vi "DAQ-AI Mean Value.vi"(8 "Cluster":T2, 11 "data":dbl[][](array[numeric]) format="%0.2f") -> ()   [LabVIEW 2015]
uses:
  <vilib>/Analysis/baseanly.llb/Mean (DBL).vi
  Galobal variable_TI.vi
  <vilib>/Analysis/NI_AALBase.lvlib
  <vilib>/ptbypt/NI_PtbyPt.lvlib
panel:
  out "element":bool
  out "Sensor Data":T1
  out "Analog":dbl[](array[numeric])
  out "AI_as DI":bool[](array[boolean])
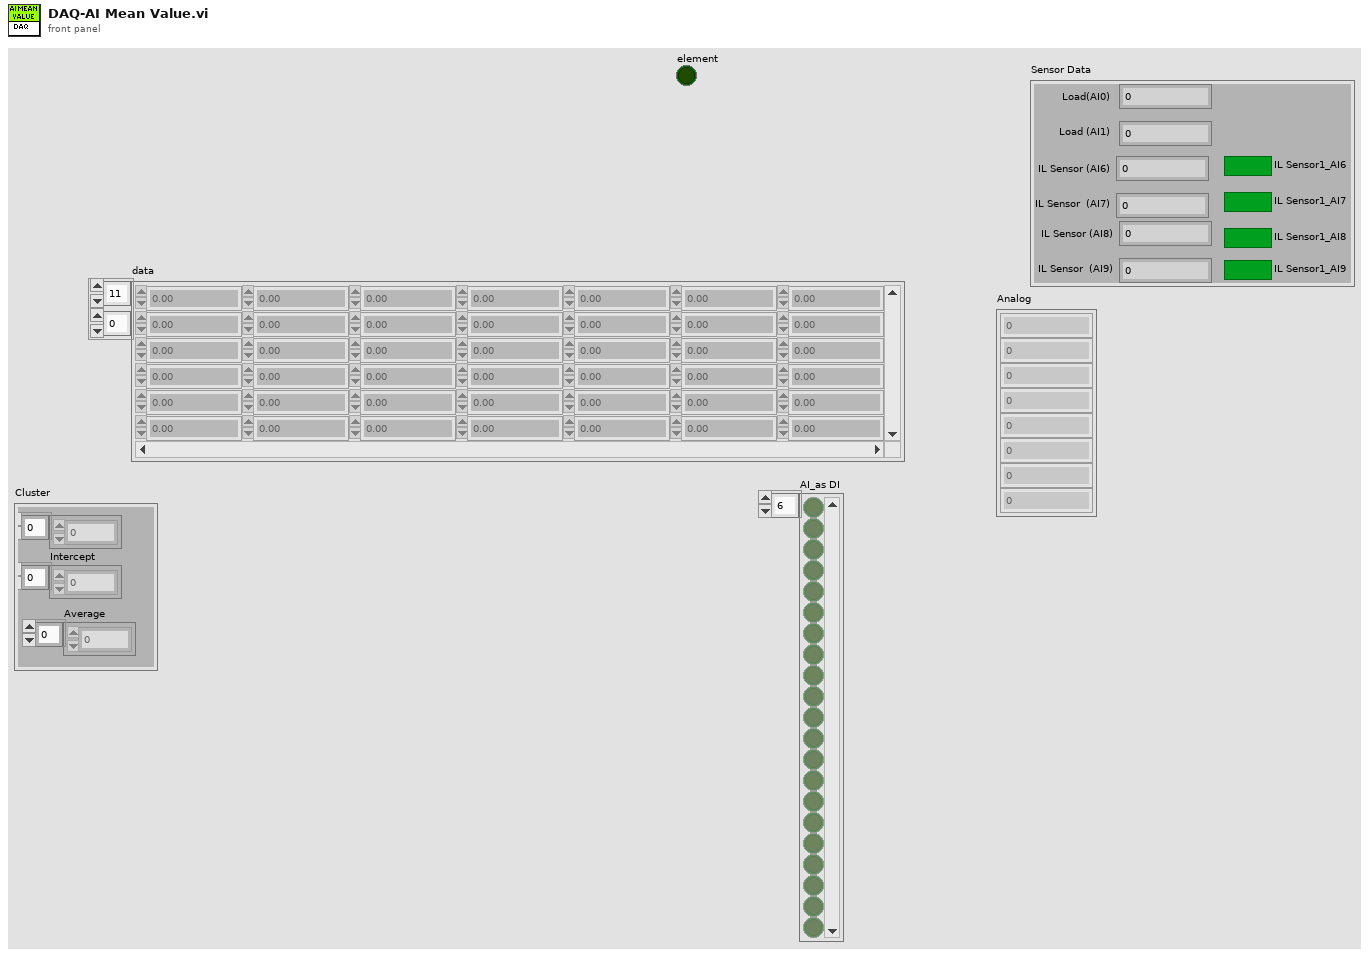
[diagram p1: front panel]
types:
  T1 = cluster{"Load(AI0) ":dbl, "Load (AI1) ":dbl, "IL Sensor (AI6)":dbl, "IL Sensor  (AI7)":dbl, "IL Sensor (AI8)":dbl, "IL Sensor  (AI9)":dbl, "IL Sensor1_AI6":bool, "IL Sensor1_AI7":bool, "IL Sensor1_AI8":bool, "IL Sensor1_AI9":bool}
  T2 = cluster{"Slop":dbl[], "Intercept":dbl[], "Average ":i16[]}
  T3 = cluster{"IL Sensor_Max (AI6)":dbl, "IL Sensor_Min (AI6)":dbl, "IL Sensor_Max (AI7)":dbl, "IL Sensor _Min (AI7)":dbl, "IL Sensor_Max (AI8)":dbl, "IL Sensor_Min (AI8)":dbl, "IL Sensor_Max  (AI9)":dbl, "IL Sensor_Min  (AI9)":dbl}
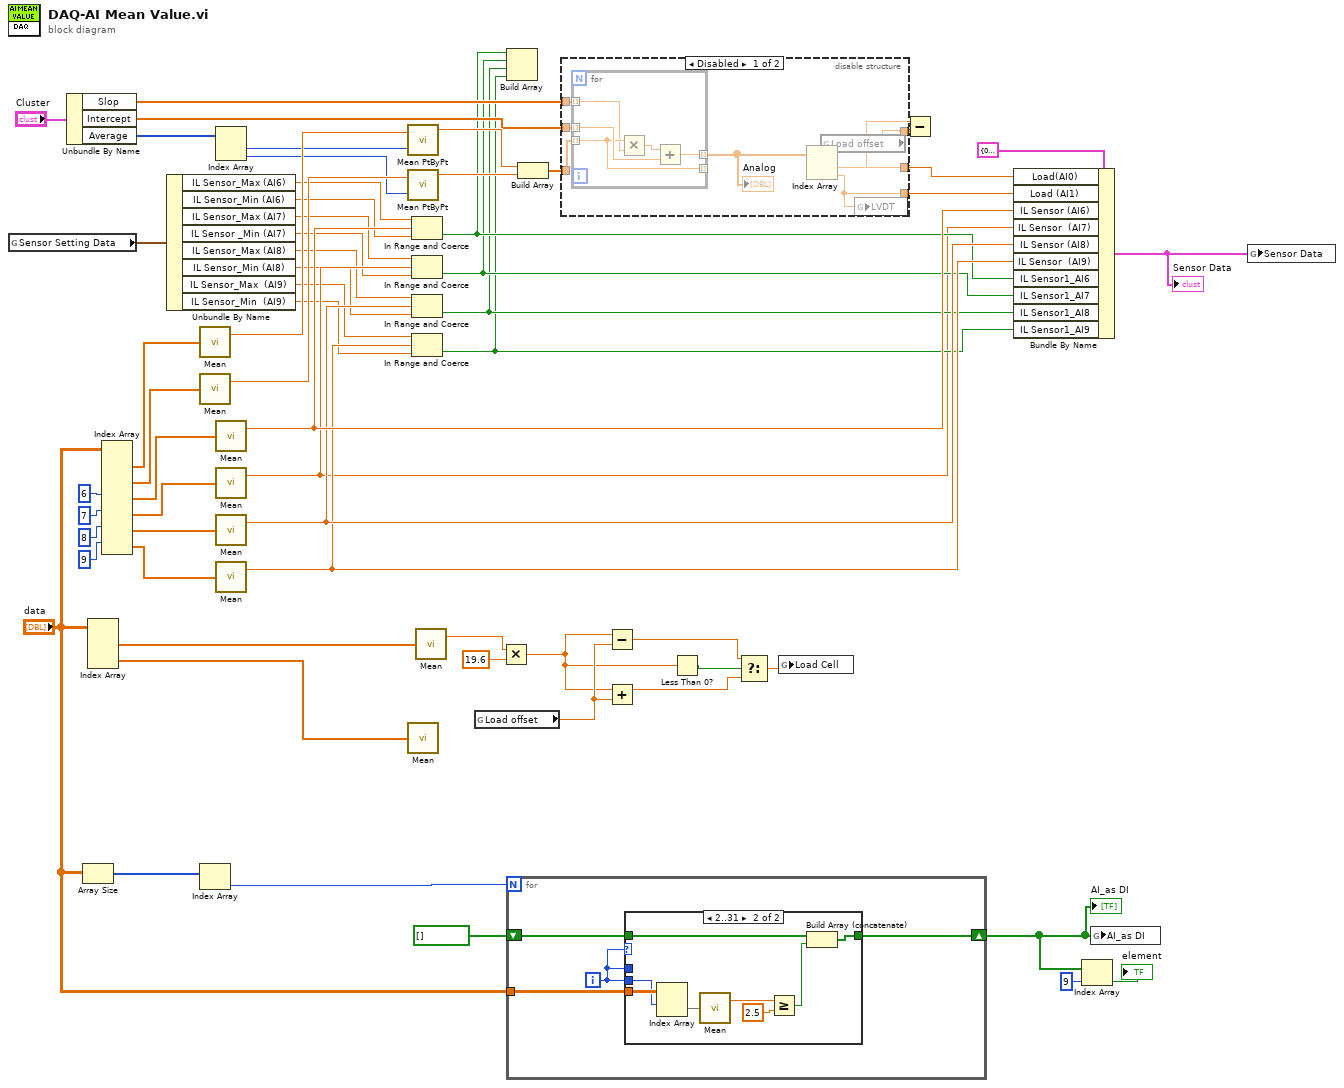
[diagram p0: block diagram]
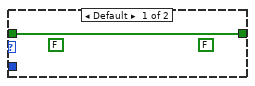
[diagram p3: hidden frame]
diagram:
  n1 = global read "Galobal variable_TI.vi" "Sensor Setting Data"() -> (w14:T3)
  n2 = Unbundle By Name("Cluster") -> ("Slop"=w45:dbl[], "Intercept"=w44:dbl[], "Average"=w43:i16[])
  n3 = Array Size(array="data") -> (size(s)=w59:i32[])
  n4 = Index Array(array="data") -> (element #1=w57:dbl[], element #2=w60:dbl[])  [unwired: 4 in]
  n5 = Index Array(array="data", index (row) #3=6 ("index (row)"), index (row) #4=7 ("index (row)"), index (row) #5=8 ("index (row)"), index (row) #6=9 ("index (row)")) -> (element #1=w48:dbl[], element #2=w47:dbl[], element #3=w35:dbl[], element #4=w42:dbl[], element #5=w37:dbl[], element #6=w36:dbl[])  [unwired: 8 in]
  n6 = Unbundle By Name(w14) -> ("IL Sensor_Max (AI6)"=w22:dbl, "IL Sensor_Min (AI6)"=w21:dbl, "IL Sensor_Max (AI7)"=w20:dbl, "IL Sensor _Min (AI7)"=w19:dbl, "IL Sensor_Max (AI8)"=w18:dbl, "IL Sensor_Min (AI8)"=w17:dbl, "IL Sensor_Max  (AI9)"=w16:dbl, "IL Sensor_Min  (AI9)"=w15:dbl)
  n7 = call-poly <vilib>:"Mean.vi"("X"=w48) -> ("mean"=w54:dbl)  [unwired: 1 out]
  n8 = call-poly <vilib>:"Mean.vi"("X"=w47) -> ("mean"=w53:dbl)  [unwired: 1 out]
  n9 = Index Array(array=w59) -> (element=w56:i32)  [unwired: 1 in]
  n10 = Index Array(array=w43) -> (element #1=w52:i16, element #2=w51:i16)  [unwired: 2 in]
  n11 = call-poly <vilib>:"Mean.vi"("X"=w35) -> ("mean"=w32:dbl)  [unwired: 1 out]
  n12 = call-poly <vilib>:"Mean.vi"("X"=w42) -> ("mean"=w23:dbl)  [unwired: 1 out]
  n13 = call-poly <vilib>:"Mean.vi"("X"=w37) -> ("mean"=w31:dbl)  [unwired: 1 out]
  n14 = call-poly <vilib>:"Mean.vi"("X"=w36) -> ("mean"=w30:dbl)  [unwired: 1 out]
  n15 = call <vilib>:"Mean PtByPt.vi"("x"=w54, "sample length"=w52) -> ("mean"=w50:dbl)  [unwired: 2 in, 1 out]
  n16 = call <vilib>:"Mean PtByPt.vi"("x"=w53, "sample length"=w51) -> ("mean"=w49:dbl)  [unwired: 2 in, 1 out]
  n17 = call-poly <vilib>:"Mean.vi"("X"=w60) -> ()  [unwired: 2 out]
  n18 = In Range and Coerce(upper limit=w22, x=w32, lower limit=w21) -> (In Range?=w28:bool)  [unwired: 1 out]
  n19 = In Range and Coerce(upper limit=w20, x=w23, lower limit=w19) -> (In Range?=w27:bool)  [unwired: 1 out]
  n20 = In Range and Coerce(upper limit=w18, x=w31, lower limit=w17) -> (In Range?=w26:bool)  [unwired: 1 out]
  n21 = In Range and Coerce(upper limit=w16, x=w30, lower limit=w15) -> (In Range?=w25:bool)  [unwired: 1 out]
  n22 = call-poly <vilib>:"Mean.vi"("X"=w57) -> ("mean"=w8:dbl)  [unwired: 1 out]
  n23 = global read "Galobal variable_TI.vi" "Load offset"() -> (w6:dbl)
  n24 = Multiply(x=w8, y=19.6) -> (x*y=w5:dbl)
  n25 = Build Array(w28, w27, w26, w25) -> ()  [unwired: 1 out]
  n26 = for {
    N: w56 -> [_]
    tunnel: "data" -> [w64]
    shift-right: [w61] -> w13
    shift-left: bool[] [] -> [w63]
    i -> [w62]
    n27 = case shown="2..31" w62 {
      tunnel: w64 -> [_ w73]
      tunnel: w62 -> [_ w69]
      tunnel: [w65 w72] -> w61
      tunnel: w63 -> [w65 w71]
      tunnel: w62 -> [_ _]
      frame Default {
        (unwired) FALSE
        (unwired) FALSE
      }
      frame 2..31 {
        n28 = Index Array(array=w73, index (row)=w69) -> (element=w67:dbl[])  [unwired: 1 in]
        n29 = call-poly <vilib>:"Mean.vi"("X"=w67) -> ("mean"=w66:dbl)  [unwired: 1 out]
        n30 = Greater Or Equal?(x=w66, y=2.5) -> (x >= y?=w68:bool)
        n31 = Build Array (concatenate)(w71, w68) -> (w72:bool[])
      }
    }
  }
  "AI_as DI" <- w13
  n32 = Build Array(w50, w49) -> (w33:dbl[])
  n33 = disable-structure shown="Disabled" {
    disable-tunnel: w45 -> [w80 _]
    disable-tunnel: w44 -> [w79 _]
    disable-tunnel: [w77 _] -> w34
    disable-tunnel: w33 -> [w76 _]
    disable-tunnel: [w75 _] -> w10
    disable-tunnel: [w74 _] -> w9
    frame Disabled {
      n34 = for {
        tunnel: w80 -> [w81] mode=indexing
        tunnel: w79 -> [w84] mode=indexing
        tunnel: w76 -> [w83] mode=indexing
        tunnel: [w83] -> _ mode=indexing
        tunnel: [w82] -> w78 mode=indexing
        n35 = Multiply(x=w83, y=w81) -> (x*y=w85:dbl)
        n36 = Add(x=w85, y=w84) -> (x+y=w82:dbl)
      }
      "Analog" <- w78
      n37 = Index Array(array=w78) -> (element #1=w75:dbl, element #2=w77:dbl)  [unwired: 2 in]
      n38 = global read "Galobal variable_TI.vi" "Load offset"() -> (w74:dbl)
      n39 = global write "Galobal variable_TI.vi" "LVDT"(w77) -> ()
    }
    frame Enabled {
    }
  }
  n40 = Subtract(x=w5, y=w6) -> (x-y=w3:dbl)
  n41 = Add(x=w5, y=w6) -> (x+y=w2:dbl)
  n42 = Less Than 0?(x=w5) -> (x < 0?=w4:bool)
  n43 = Select(t=w3, s=w4, f=w2) -> (s? t:f=w1:dbl)
  n44 = global write "Galobal variable_TI.vi" "Load Cell"(w1) -> ()
  n45 = Subtract(x=w10, y=w9) -> ()  [unwired: 1 out]
  n46 = Bundle By Name(cluster=T1 {"Load(AI0) "=0.0, "Load (AI1) "=0.0, "IL Sensor (AI6)"=0.0, "IL Sensor  (AI7)"=0.0, "IL Sensor (AI8)"=0.0, "IL Sensor  (AI9)"=0.0, "IL Sensor1_AI6"=FALSE, "IL Sensor1_AI7"=FALSE, "IL Sensor1_AI8"=FALSE, "IL Sensor1_AI9"=FALSE} ("Sensor Data"), "Load(AI0)"=w10, "Load (AI1)"=w34, "IL Sensor (AI6)"=w32, "IL Sensor  (AI7)"=w23, "IL Sensor (AI8)"=w31, "IL Sensor  (AI9)"=w30, "IL Sensor1_AI6"=w28, "IL Sensor1_AI7"=w27, "IL Sensor1_AI8"=w26, "IL Sensor1_AI9"=w25) -> (w24:T1)
  "Sensor Data" <- w24
  n47 = Index Array(array=w13, index=9) -> (element=→"element":bool)
  n48 = global write "Galobal variable_TI.vi" "AI_as DI"(w13) -> ()
  n49 = global write "Galobal variable_TI.vi" "Sensor Data"(w24) -> ()
